vi "MouseCoordsToMeters-MasterControl.vi"(2 "Picture Control Ref":refnum<vi>, 3 "Mouse Pos":cluster{"x":dbl, "y":dbl}, 4 "Arena Pixel Dim":i32[](array[numeric])) -> (0 "y (m)":dbl, 1 "x (m)":dbl)   [LabVIEW 2015, in "MissionControl2017.lvlib"]
uses:
  MissionControl2017.lvlib
  Navigation2017.lvlib
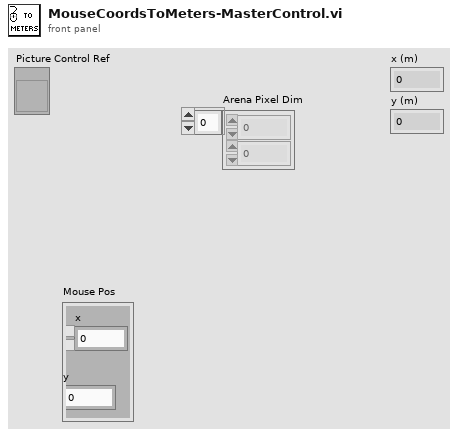
[diagram p1: front panel]
types:
  T1 = typedef "LVPositionTypeDef.ctl" = cluster{"Left":i32, "Top":i32}
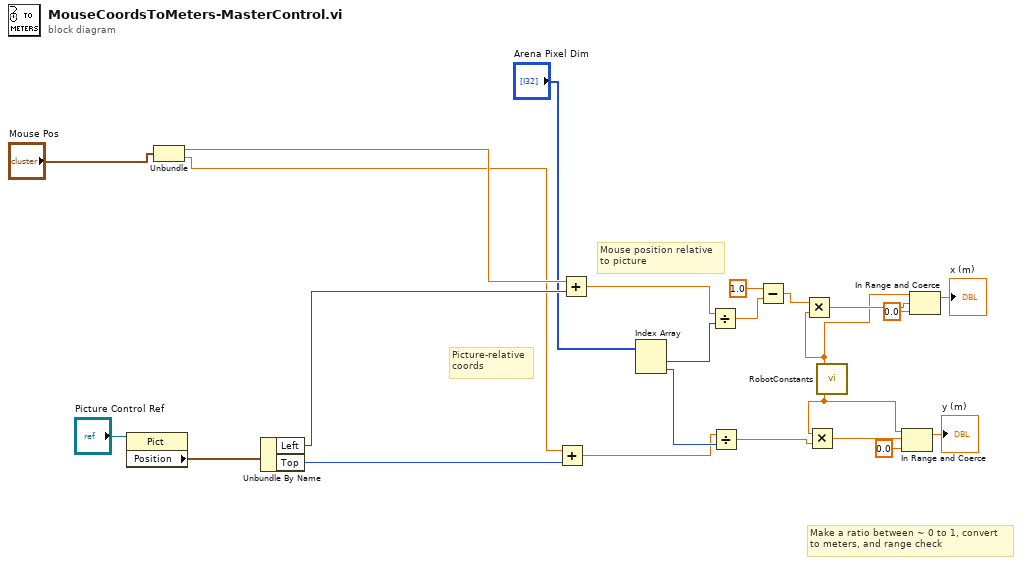
[diagram p0: block diagram]
diagram:
  # "Make a ratio between ~ 0 to 1, convert\nto meters, and range check"
  # "Mouse position relative\nto picture"
  # "Picture-relative\ncoords"
  n1 = property class="Pict"(reference="Picture Control Ref") -> ("Position"=w23:T1)  [unwired: 1 in, 2 out]
  n2 = Unbundle("Mouse Pos") -> ("x"=w19:dbl, "y"=w18:dbl)
  n3 = Unbundle By Name(w23) -> ("Left"=w21:i32, "Top"=w22:i32)
  n4 = Add(x=w18, y=w22) -> (x+y=w13:dbl)
  n5 = Add(x=w19, y=w21) -> (x+y=w15:dbl)
  n6 = Index Array(array="Arena Pixel Dim") -> (element #1=w16:i32, element #2=w14:i32)  [unwired: 2 in]
  n7 = Divide(x=w15, y=w16) -> (x/y=w3:dbl)
  n8 = Divide(x=w13, y=w14) -> (x/y=w12:dbl)
  n9 = Subtract(x=1.0, y=w3) -> (x-y=w2:dbl)
  n10 = call "RobotConstants.vi"() -> ("Arena Width (m)"=w6:dbl, "Arena Height (m)"=w7:dbl)  [unwired: 3 out]
  n11 = Multiply(x=w2, y=w6) -> (x*y=w11:dbl)
  n12 = Multiply(x=w7, y=w12) -> (x*y=w10:dbl)
  n13 = In Range and Coerce(upper limit=w7, x=w10, lower limit=0.0) -> (coerced(x)=→"y (m)":dbl)  [unwired: 1 out]
  n14 = In Range and Coerce(upper limit=w6, x=w11, lower limit=0.0) -> (coerced(x)=→"x (m)":dbl)  [unwired: 1 out]
